vi "SCPI_write_volt.vi"() -> ()   [LabVIEW 2020]
doc: "Wysyłanie podstawowych komend SCPI - zasilacz SIGLENT SPD3303X-E"
panel:
  in  "stop":bool
  out "Waveform Chart":dbl(graph)
  out "error out":errorcluster
  in  "CH1 / CH2":bool
  in  "VOLT / CURR":bool
  in  "Knob":dbl(knob) scale=0.0..10.0
  in  "VISA resource name":refnum<visa-resource-name>
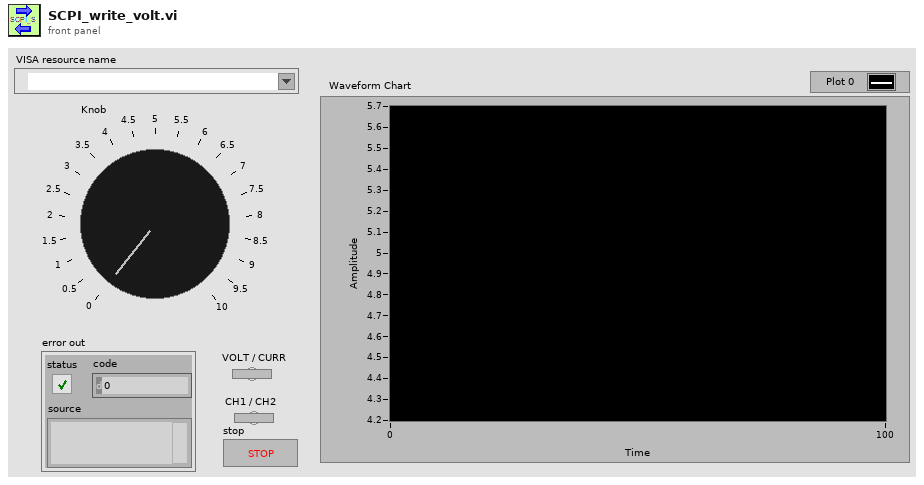
[diagram p1: front panel]
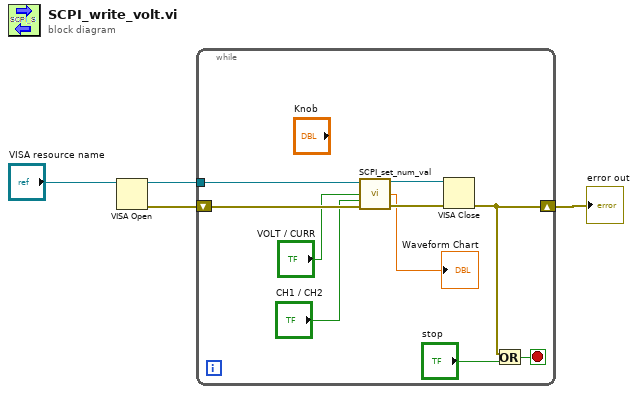
[diagram p0: block diagram]
diagram:
  n1 = VISA Open(VISA resource name="VISA resource name") -> (VISA resource name=w3:refnum<visa-resource-name>, error out=w2:errorcluster)  [unwired: 4 in]
  n2 = while {
    tunnel: w3 -> [w14]
    shift-right: [w6] -> w1
    shift-left: w2 -> [w13]
    stop <- w7 stop-if-true
    n3 = call "SCPI_set_num_val.vi"("VISA"=w14, "Volt / Curr"="VOLT / CURR", "CH1/CH2"="CH1 / CH2", "error in (no error)"=w13) -> ("VISA resource name out"=w10:refnum<visa-resource-name>, "numeric value"=→"Waveform Chart":dbl, "error out"=w9:errorcluster)  [unwired: 9 in]
    n4 = VISA Close(VISA resource name=w10, error in (no error)=w9) -> (error out=w6:errorcluster)
    n5 = Or(x=w6, y="stop") -> (x .or. y?=w7:bool)
  }
  "error out" <- w1
